vi "createImage.vi"(8 "error in (no error)":errorcluster, 9 "ImageName":string, 10 "imageString":string, 11 "ImageAnalyser in":refnum<class "ImageAnalyser.lvclass">) -> (0 "error out":errorcluster, 2 "ImageData":T1, 3 "ImageAnalyser out":refnum<class "ImageAnalyser.lvclass">)   [LabVIEW 2011, in "Tools.lvlib" / "Imaging.lvlib" / "ImageAnalyser.lvclass"]
uses:
  ImageAnalyser.lvclass
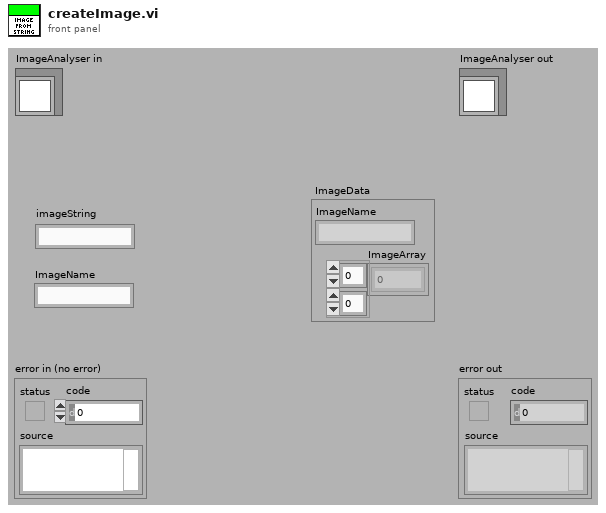
[diagram p1: front panel]
types:
  T1 = cluster{"ImageName":string, "ImageArray":dbl[][]}
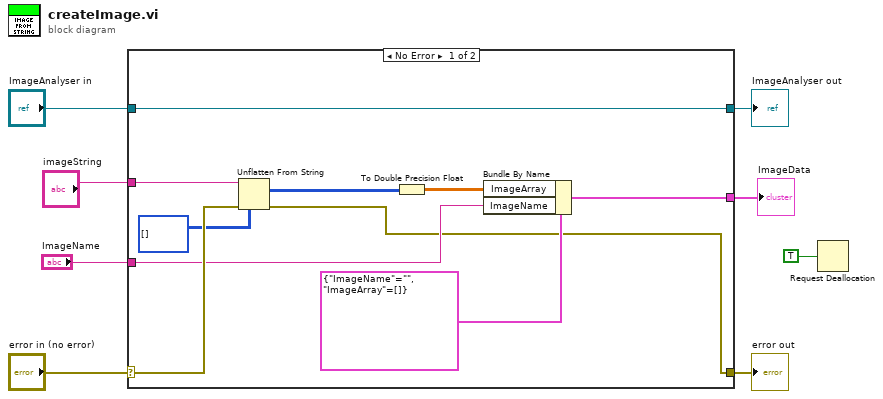
[diagram p0: block diagram]
diagram:
  n1 = case shown="No Error" "error in (no error)" {
    selector: "error in (no error)" -> [w16 w20]
    tunnel: [w11 w20] -> w7
    tunnel: [w18 w19] -> w5
    tunnel: "ImageAnalyser in" -> [w18 w19]
    tunnel: "imageString" -> [w17 _]
    tunnel: "ImageName" -> [w13 _]
    tunnel: [w12 _] -> w2
    frame No Error {
      n2 = Unflatten From String(type=u16[][] [] ("Image data"), binary string=w17, error in (no error)=w16) -> (value=w9:u16[][], error out=w11:errorcluster)  [unwired: 2 in, 1 out]
      n3 = To Double Precision Float(number=w9) -> (double precision float=w10:dbl[][])
      n4 = Bundle By Name(cluster=T1 {"ImageName"="", "ImageArray"=[]}, "ImageArray"=w10, "ImageName"=w13) -> (w12:T1)
    }
    frame Error {
    }
  }
  "error out" <- w7
  "ImageAnalyser out" <- w5
  "ImageData" <- w2
  n5 = Request Deallocation(TRUE ("flag")) -> ()
